vi "write_serial_cmd.vi"(6 "pulse duration (ms)":i32, 8 "error in":errorcluster, 9 "pressure set (mBar)":dbl, 10 "pressure command":T1, 11 "Pressure Box COM":refnum<visa-resource-name>) -> (0 "error out":errorcluster, 3 "Pressure Box COM out":refnum<visa-resource-name>)   [LabVIEW 2019]
uses:
  controls/proportionAir_cmds.ctl
  <vilib>/Instr/_visa.llb/VISA Flush IO Buffer Mask.ctl
panel:
  out "Response":string
  # "PROPORTIONAIR REGULATOR"
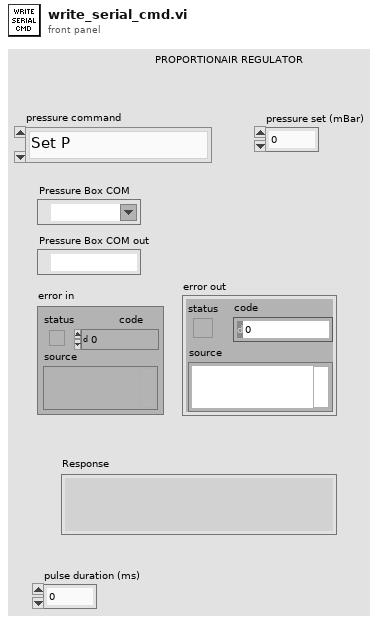
[diagram p1: front panel]
types:
  T1 = typedef "proportionAir_cmds.ctl" = enum16{"Set P", "Switch to Atm", "Switch to Regulator", "Pulse", "WC"}
  T2 = typedef "VISA Flush IO Buffer Mask.ctl" = u16
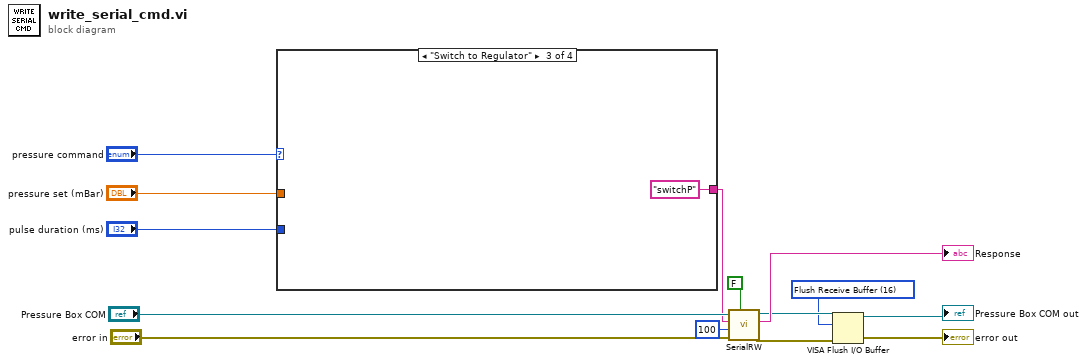
[diagram p0: block diagram]
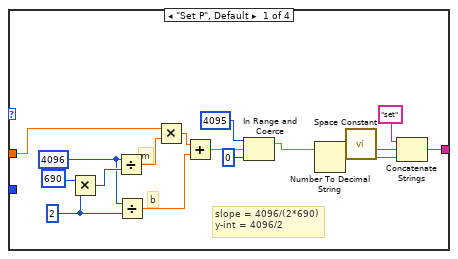
[diagram p2: hidden frame]
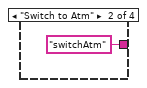
[diagram p3: hidden frame]
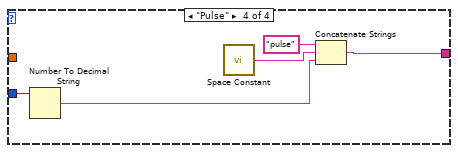
[diagram p4: hidden frame]
diagram:
  w1 = T2 16 items=["Flush Receive Buffer"=16, "Write Transmit Buffer to Device"=32, "Flush Receive Buffer (No I/O)"=64, "Flush Transmit Buffer"=128] ("Mask")
  n1 = case shown="\"Switch to Regulator\"" "pressure command" {
    tunnel: "pressure set (mBar)" -> [w15 _ _ _]
    tunnel: [w27 "switchAtm" "switchP" w35] -> w8
    tunnel: "pulse duration (ms)" -> [_ _ _ w36]
    frame "Set P", Default {
      w23 = 2 ("y")
      w24 = 4096
      # "b"
      # "m"
      # "slope = 4096/(2*690)\ny-int = 4096/2"
      n2 = Multiply(x=690, y=w23) -> (x*y=w25:i32)
      n3 = Divide(x=w24, y=w25) -> (x/y=w22:dbl)
      n4 = Divide(x=w24, y=w23) -> (x/y=w21:dbl)
      n5 = Multiply(x=w15, y=w22) -> (x*y=w20:dbl)
      n6 = Add(x=w20, y=w21) -> (x+y=w19:dbl)
      n7 = In Range and Coerce(upper limit=4095, x=w19, lower limit=0) -> (coerced(x)=w16:dbl)  [unwired: 1 out]
      n8 = Number To Decimal String(number=w16) -> (decimal integer string=w28:string)  [unwired: 1 in]
      n9 = call <vilib>:"Space Constant.vi"() -> ("String"=w30:string)
      n10 = Concatenate Strings("set" ("string"), w30, w28) -> (w27:string)
    }
    frame "Switch to Atm" {
    }
    frame "Switch to Regulator" {
    }
    frame "Pulse" {
      n11 = Number To Decimal String(number=w36) -> (decimal integer string=w33:string)  [unwired: 1 in]
      n12 = call <vilib>:"Space Constant.vi"() -> ("String"=w34:string)
      n13 = Concatenate Strings("pulse" ("string"), w34, w33) -> (w35:string)
    }
  }
  n14 = call "SerialRW.vi"("Query?"=FALSE, "error in (no error)"="error in", "Delay (ms)"=u32 100, "Command"=w8, "VISA handle"="Pressure Box COM") -> ("error out"=w4:errorcluster, "Response"=→"Response":string, "Dup. VISA handle"=w5:refnum<visa-resource-name>)  [unwired: 1 in, 1 out]
  n15 = VISA Flush I/O Buffer(VISA resource name=w5, mask (16)=w1, error in (no error)=w4) -> (VISA resource name out=→"Pressure Box COM out":refnum<visa-resource-name>, error out=→"error out":errorcluster)
